vi "Render Draw Line.vi"(4 "y2":i32, 6 "x2":i32, 8 "error in":errorcluster, 9 "y1":i32, 10 "x1":i32, 11 "Renderer Pointer":u32 format="%.0x") -> (0 "error out":errorcluster, 3 "Return":i32)   [LabVIEW 2015, in "LibSDL2.lvlib"]
uses:
  LibSDL2.lvlib
  DLL/SDL2.dll
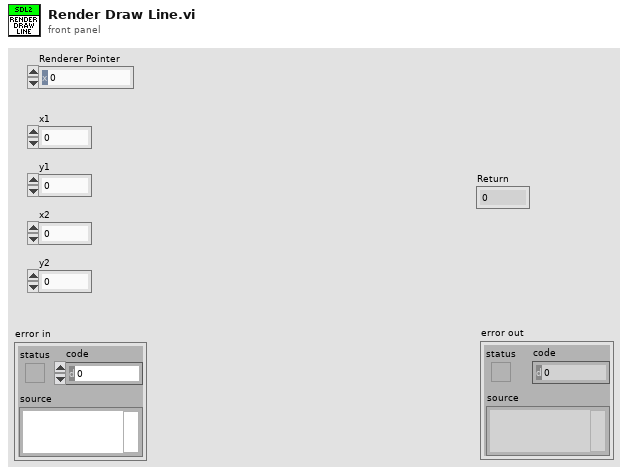
[diagram p1: front panel]
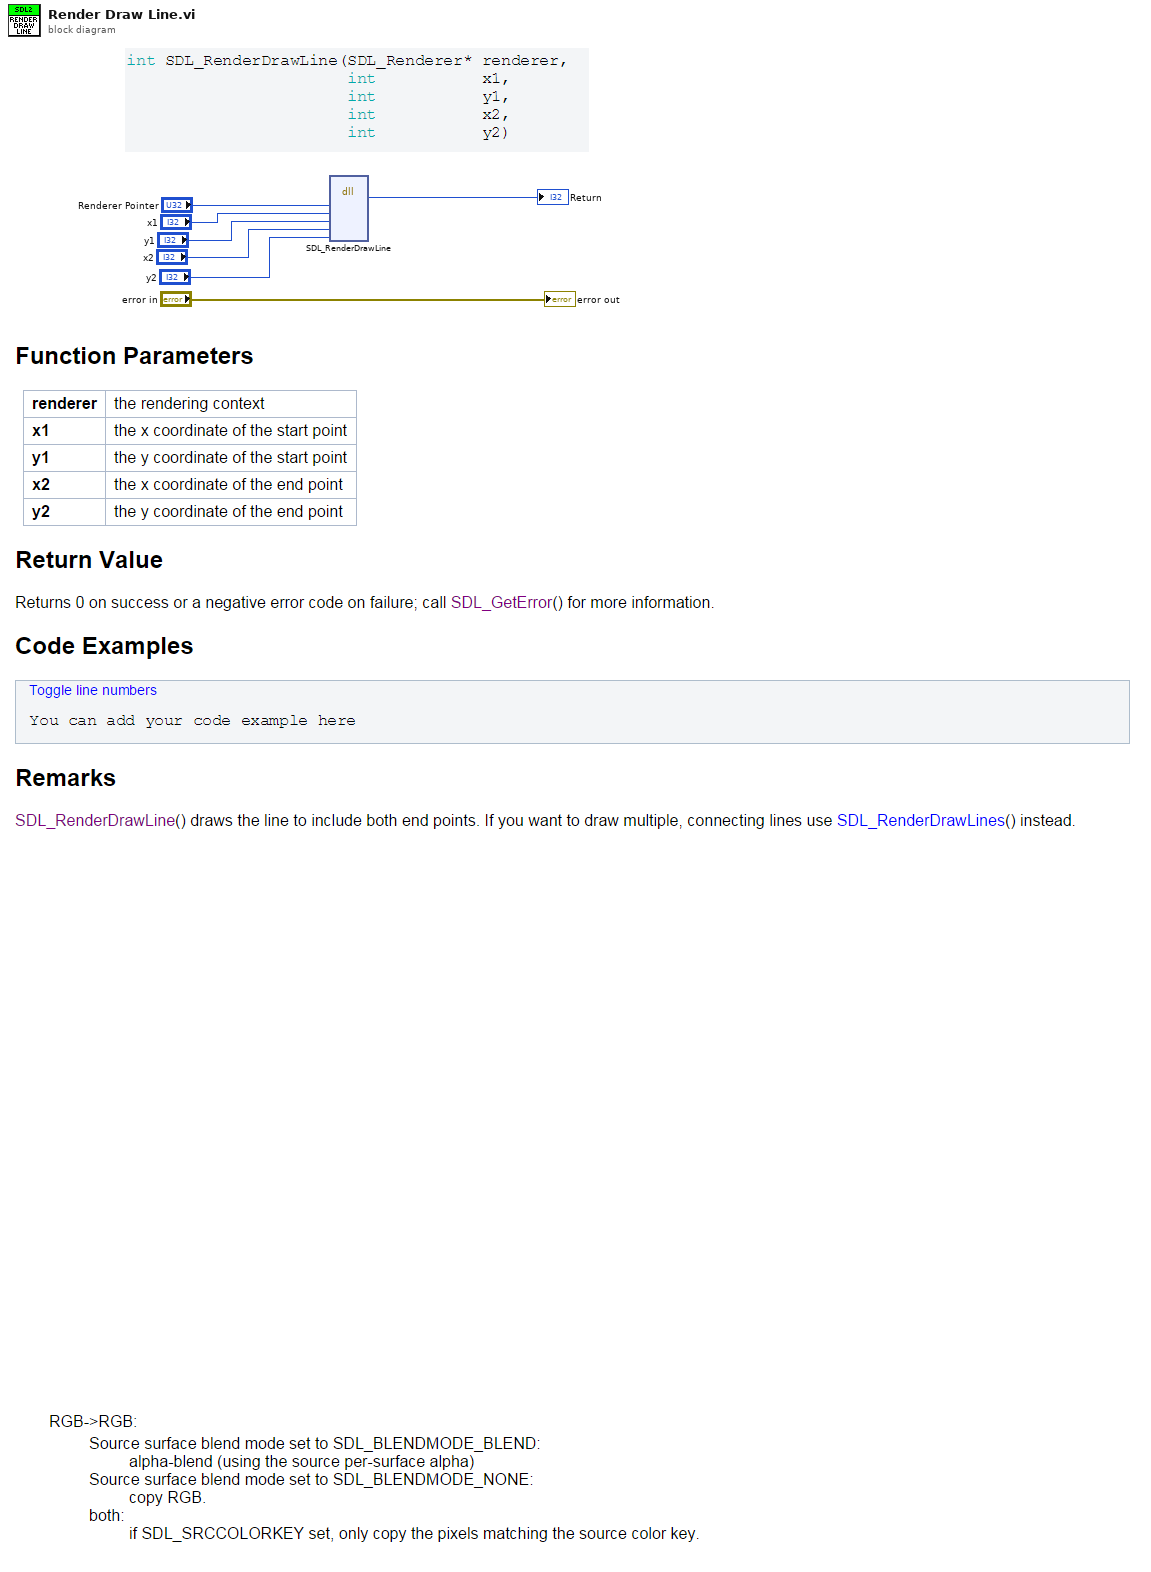
[diagram p0: block diagram]
diagram:
  n1 = dll-call lib="C:/dev/PGS/LabSDL2/Source/Libraries/LibSDL2 Wrapper/DLL/SDL2.dll" fn="SDL_RenderDrawLine"("renderer_pointer"="Renderer Pointer", "x1"="x1", "y1"="y1", "x2"="x2", "y2"="y2") -> ("return type"=→"Return":i32)  [unwired: 8 in, 2 out]
  "error out" <- "error in"
